vi "Etalonnage.vi"(7 "Reference Cell":i32=1, 8 "error in":errorcluster, 10 "Over":bool=TRUE, 11 "NextStep":bool=TRUE) -> (0 "error out":errorcluster, 1 "Résidu":dbl, 2 "CoeffsPoly":dbl[](array[numeric]), 3 "Values":cluster{dbl[], dbl[]})   [LabVIEW 2013]
uses:
  GlobalVariables/CalibrationVolumes.vi
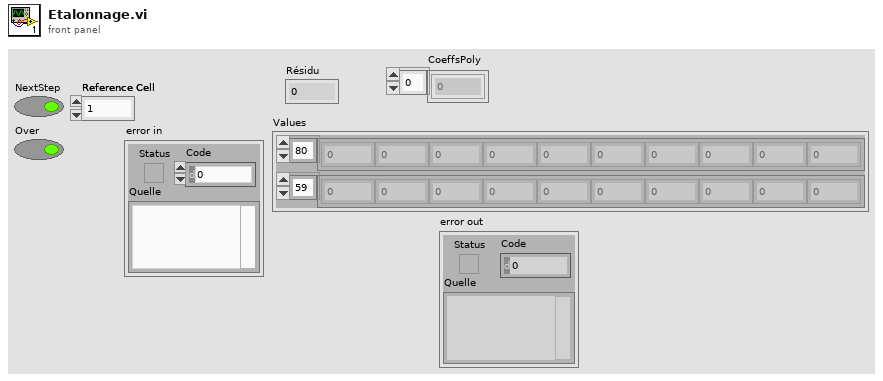
[diagram p1: front panel]
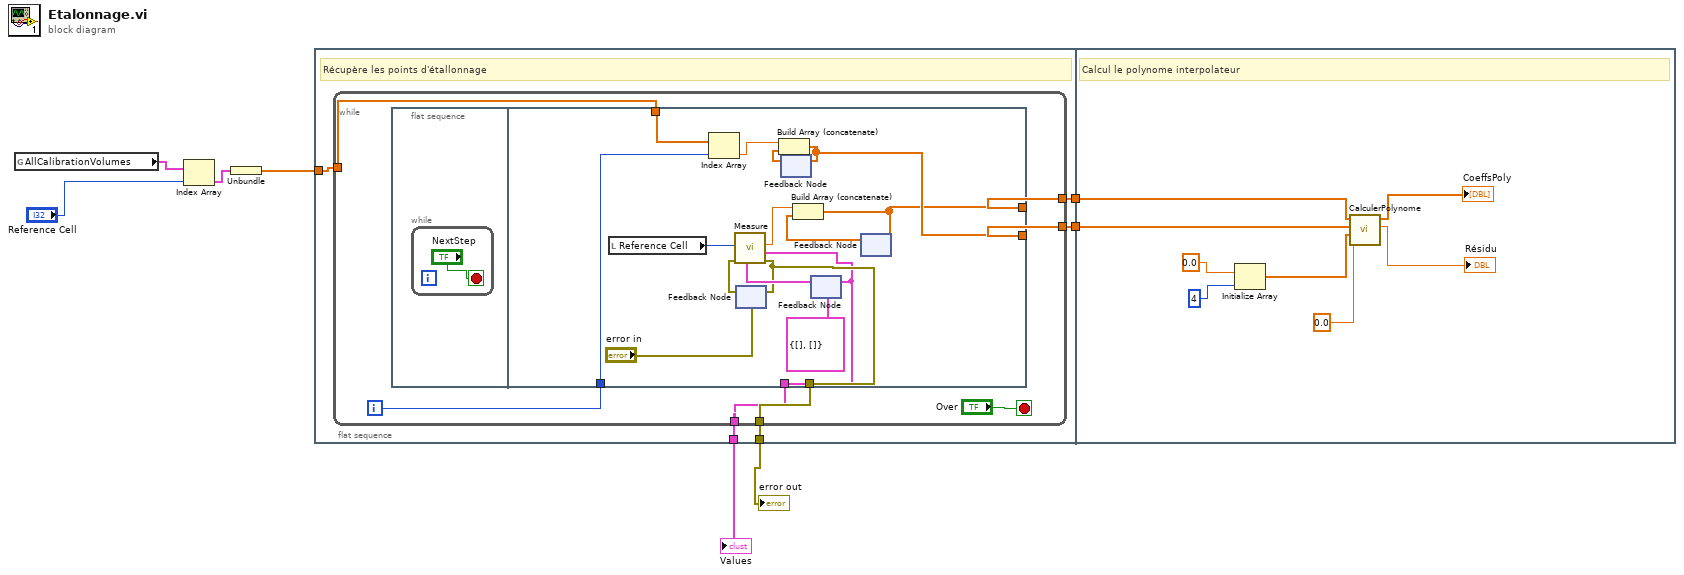
[diagram p0: block diagram]
diagram:
  n1 = global read "CalibrationVolumes.vi" "AllCalibrationVolumes"() -> (w4:cluster{"CalibrationVolumes":dbl[]}[])
  n2 = Index Array(array=w4, index="Reference Cell") -> (element=w2:cluster{"CalibrationVolumes":dbl[]})
  n3 = Unbundle(w2) -> ("CalibrationVolumes"=w1:dbl[])
  n4 = flat-sequence {
    tunnel: [w13] -> w8
    tunnel: [w12] -> w7
    tunnel: [w11] -> w6
    tunnel: [w10] -> w5
    tunnel: w1 -> [w9]
    tunnel: w8 -> [w44]
    tunnel: w7 -> [w43]
    frame #0 {
      # "Récupère les points d'étallonnage"
      n5 = while {
        tunnel: [w19] -> w10
        tunnel: [w18] -> w13
        tunnel: [w17] -> w12
        tunnel: [w16] -> w11
        tunnel: w9 -> [w14]
        i -> [w15]
        stop <- "Over" stop-if-true
        n6 = flat-sequence {
          tunnel: [w29] -> w19
          tunnel: [w28] -> w18
          tunnel: [w27] -> w17
          tunnel: [w26] -> w16
          tunnel: w15 -> [w24]
          tunnel: w14 -> [w22]
          frame #0 {
            n7 = while {
              stop <- "NextStep" stop-if-true
            }
          }
          frame #1 {
            n8 = local read "Reference Cell"() -> (w23:i32)
            n9 = Index Array(array=w22, index=w24) -> (element=w25:dbl)
            n10 = feedback #1("error in") -> (w36:errorcluster)
            n11 = feedback #2() -> (w30:dbl[])  [unwired: 1 in]
            n12 = Build Array (concatenate)(w25, w30) -> (w28:dbl[])
            n13 = feedback-in #2(w28) -> ()
            n14 = feedback #3(cluster{dbl[], dbl[]} {[], []} ("Graph in")) -> (w35:cluster{dbl[], dbl[]})
            n15 = call "Measure.vi"("Graph in"=w35, "error in"=w36, "Reference Cell"=w23) -> ("error out"=w29:errorcluster, "Values"=w26:cluster{dbl[], dbl[]}, "P1/P2"=w34:dbl)  [unwired: 6 in]
            n16 = feedback-in #1(w29) -> ()
            n17 = feedback-in #3(w26) -> ()
            n18 = feedback #4() -> (w33:dbl[])  [unwired: 1 in]
            n19 = Build Array (concatenate)(w34, w33) -> (w27:dbl[])
            n20 = feedback-in #4(w27) -> ()
          }
        }
      }
    }
    frame #1 {
      # "Calcul le polynome interpolateur"
      n21 = Initialize Array(0.0, 4) -> (w40:dbl[])
      n22 = call "CalculerPolynome.vi"("e3 [in]"=0.0, "Meilleure poly [in]"=w40, "Y"=w44, "X"=w43) -> ("Résidu [out]"=→"Résidu":dbl, "Meilleur poly [out]"=→"CoeffsPoly":dbl[])  [unwired: 6 in]
    }
  }
  "Values" <- w6
  "error out" <- w5
